vi "Startup.vi"   [LabVIEW 2016, in "Assert API Components.lvlib"]
uses:
  Assert API Components/Assert API Components.lvlib
  Assert Startup UI/Assert Startup UI/Assert Startup UI.lvclass
  C:/Program Files (x86)/National Instruments/LabVIEW 2016/vi.lib/ActorFramework/Actor/Actor.lvclass
  <vilib>/ActorFramework/Actor/Actor.lvclass
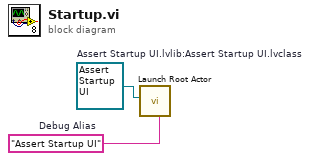
[diagram p0: block diagram]
diagram:
  w1 = "Assert Startup UI"  # Debug Alias
  w2 = refnum<class "Assert Startup UI.lvclass"> refnum  # Assert Startup UI.lvlib:Assert Startup UI.lvclass
  n1 = call <vilib>:"Launch Root Actor.vi"("Debug Alias"=w1, "Actor"=w2) -> ()  [unwired: 8 in, 2 out]
